vi "testTcpServerBase.vi"(8 "error in (no error)":errorcluster) -> (0 "error out":errorcluster)   [LabVIEW 2018]
doc: "Test TcpServerBase class."
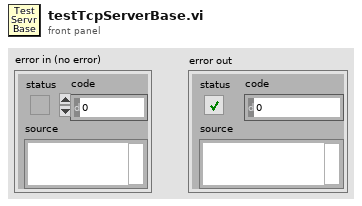
[diagram p1: front panel]
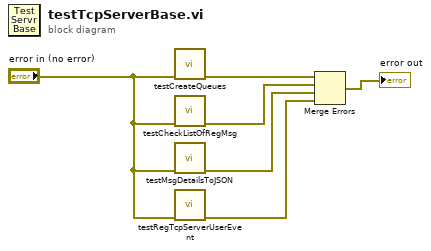
[diagram p0: block diagram]
diagram:
  n1 = call "testCreateQueues.vi"("error in (no error)"="error in (no error)") -> ("error out"=w5:errorcluster)  [unwired: 10 in]
  n2 = call "testCheckListOfRegMsg.vi"("error in (no error)"="error in (no error)") -> ("error out"=w4:errorcluster)  [unwired: 10 in]
  n3 = call "testMsgDetailsToJSON.vi"("error in (no error)"="error in (no error)") -> ("error out"=w3:errorcluster)  [unwired: 10 in]
  n4 = call "testRegTcpServerUserEvent.vi"("error in (no error)"="error in (no error)") -> ("error out"=w2:errorcluster)  [unwired: 10 in]
  n5 = Merge Errors(w5, w4, w3, w2) -> (→"error out":errorcluster)
